vi "Scripting_ConnecorPaneCreateConstant.vi"(0 "ViRef":refnum<vi>, 1 "SubViThatHasChangedConnectorPane":path, 2 "ConnectorPaneIndexToCReateConstantsOn":u32[](array[numeric]), 5 "error in (no error)":errorcluster) -> (19 "error out":errorcluster)   [LabVIEW 2014]
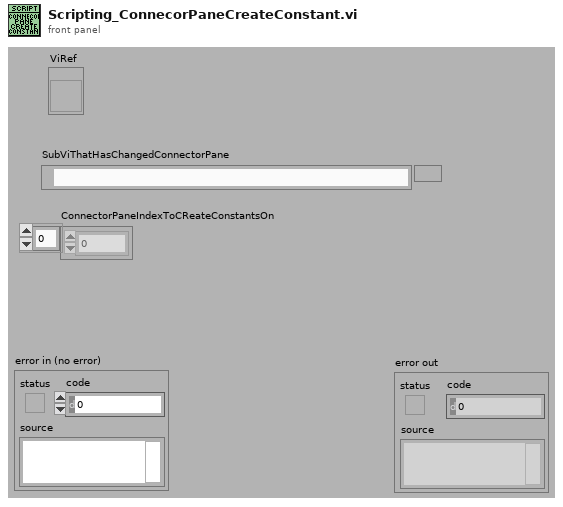
[diagram p1: front panel]
types:
  T1 = cluster{"New":refnum<vi>, "Terminals[]":refnum<vi>[]}
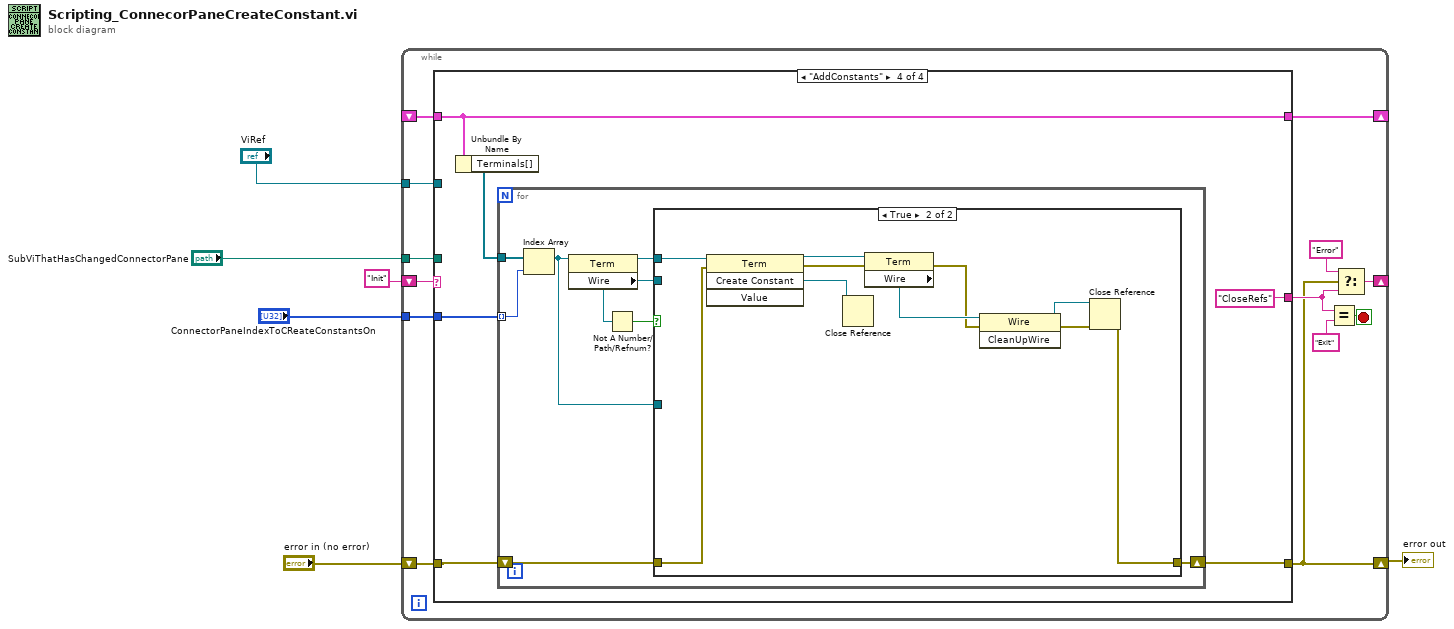
[diagram p0: block diagram]
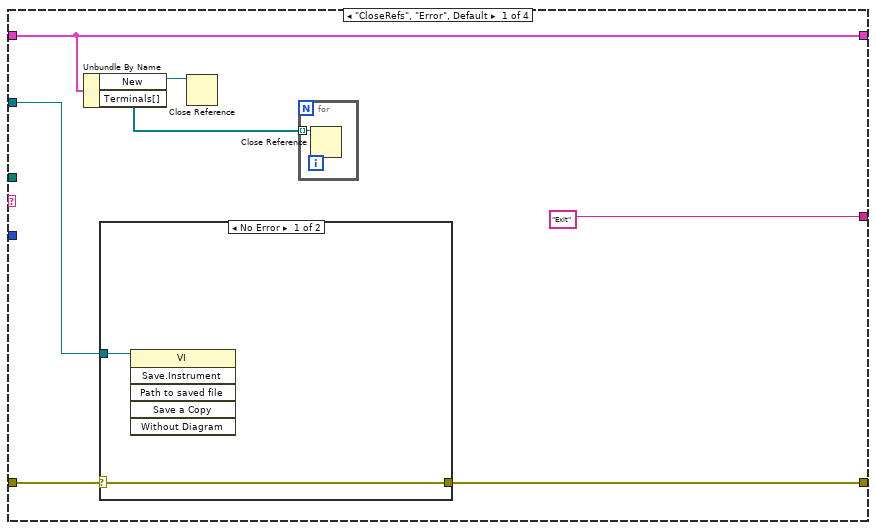
[diagram p2: hidden frame]
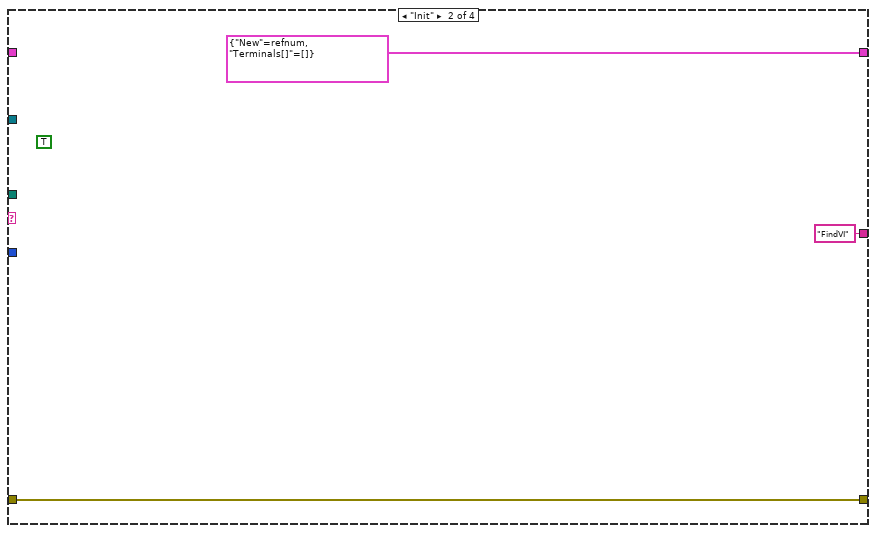
[diagram p4: hidden frame]
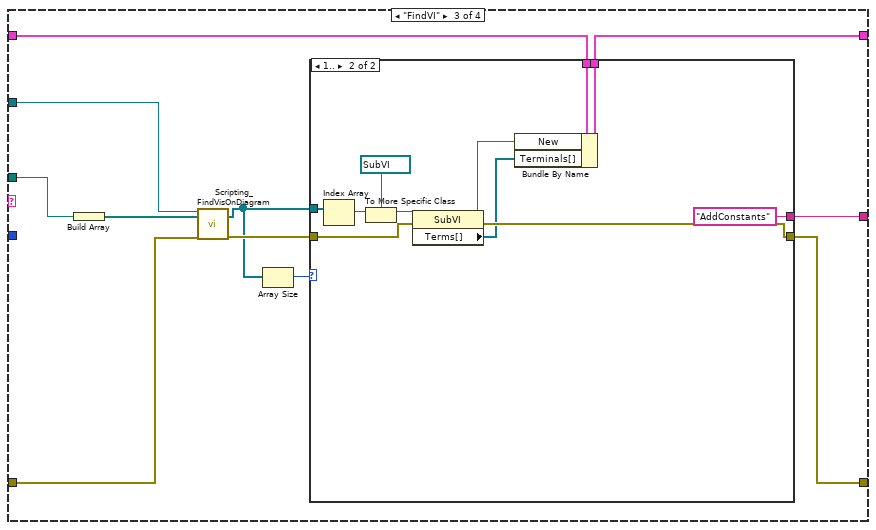
[diagram p5: hidden frame]
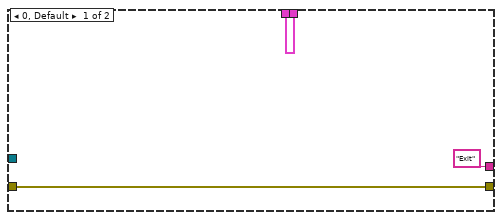
[diagram p6: hidden frame]
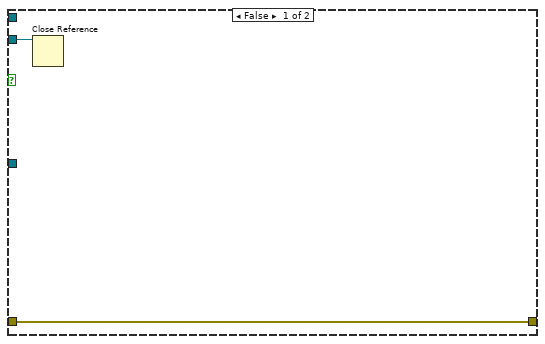
[diagram p7: hidden frame]
diagram:
  n1 = while {
    shift-right: [w12] -> w4
    shift-left: "error in (no error)" -> [w19]
    shift-right: [w17] -> _
    shift-left: "Init" -> [w18]
    shift-right: [w11] -> _
    shift-left: _ -> [w10]
    tunnel: "ViRef" -> [w9]
    tunnel: "SubViThatHasChangedConnectorPane" -> [w8]
    tunnel: "ConnectorPaneIndexToCReateConstantsOn" -> [w7]
    stop <- w16 stop-if-true
    n2 = case shown="\"AddConstants\"" w18 {
      tunnel: w19 -> [w24 w32 w43 w60]
      tunnel: [w23 w32 w35 w59] -> w12
      tunnel: ["Exit" "FindVI" w34 "CloseRefs"] -> w13
      tunnel: [w25 T1 {"New"=refnum, "Terminals[]"=[]} w38 w64] -> w11
      tunnel: w10 -> [w25 _ w39 w64]
      tunnel: w9 -> [w22 _ w42 _]
      tunnel: w8 -> [_ _ w41 _]
      tunnel: w7 -> [_ _ _ w61]
      frame "CloseRefs", "Error", Default {
        n3 = Unbundle By Name(w25) -> ("New"=w20:refnum<vi>, "Terminals[]"=w21:refnum<vi>[])
        n4 = case shown="No Error" w24 {
          selector: w24 -> [w28 w30]
          tunnel: [w28 w30] -> w23
          tunnel: w22 -> [w29 _]
          frame No Error {
            n5 = invoke class="VI" method="Save.Instrument"(reference=w29) -> ()  [unwired: 5 in, 6 out]
          }
          frame Error {
          }
        }
        n6 = Close Reference(reference=w20) -> ()  [unwired: 1 in, 1 out]
        n7 = for {
          tunnel: w21 -> [w27] mode=indexing
          n8 = Close Reference(reference=w27) -> ()  [unwired: 1 in, 1 out]
        }
      }
      frame "Init" {
        (unwired) TRUE ("Execution:Is Reentrant")
      }
      frame "FindVI" {
        n9 = Build Array(w41) -> (w40:path[])
        n10 = call <resource>:"Scripting_FindVisOnDiagram.vi"("ViRef"=w42, "VIsToSerachFor/ViName"=w40, "error in (no error)"=w43) -> ("VisFound"=w37:refnum<vi>[], "error out"=w44:errorcluster)  [unwired: 15 in]
        n11 = Array Size(array=w37) -> (size(s)=w36:i32)
        n12 = case shown="1.." w36 {
          tunnel: w44 -> [w46 w56]
          tunnel: w39 -> [w47 w54]
          tunnel: [w47 w53] -> w38
          tunnel: w37 -> [_ w52]
          tunnel: [w46 w51] -> w35
          tunnel: ["Exit" "AddConstants"] -> w34
          frame 0, Default {
          }
          frame 1.. {
            n13 = Index Array(array=w52) -> (element=w58:refnum<vi>)  [unwired: 1 in]
            n14 = To More Specific Class(target class=refnum<vi> refnum ("WhileLoop"), reference=w58) -> (specific class reference=w57:refnum<vi>)  [unwired: 1 in, 1 out]
            n15 = property class="SubVI"(reference=w57, error in=w56) -> (reference out=w50:refnum<vi>, error out=w51:errorcluster, "Terms[]"=w49:refnum<vi>[])
            n16 = Bundle By Name(cluster=w54, "New"=w50, "Terminals[]"=w49) -> (w53:T1)
          }
        }
      }
      frame "AddConstants" {
        n17 = Unbundle By Name(w64) -> ("Terminals[]"=w62:refnum<vi>[])
        n18 = for {
          tunnel: w62 -> [w68]
          tunnel: w61 -> [w72] mode=indexing
          shift-right: [w70] -> w59
          shift-left: w60 -> [w71]
          n19 = Index Array(array=w68, index=w72) -> (element=w69:refnum<vi>)
          n20 = property class="Term"(reference=w69) -> (reference out=w66:refnum<vi>, "Wire"=w65:refnum<vi>)  [unwired: 1 in, 1 out]
          n21 = Not A Number/Path/Refnum?(number/path/refnum=w65) -> (NaN/Path/Refnum?=w67:bool)
          n22 = case shown="True" w67 {
            tunnel: w71 -> [w74 w76]
            tunnel: [w74 w81] -> w70
            tunnel: w69 -> [_ _]
            tunnel: w66 -> [_ w80]
            tunnel: w65 -> [w73 _]
            frame False {
              n23 = Close Reference(reference=w73) -> ()  [unwired: 1 in, 1 out]
            }
            frame True {
              n24 = invoke class="Term" method="Create Constant"(reference=w80, error in=w76) -> (reference out=w79:refnum<vi>, error out=w78:errorcluster, "Create Constant"=w75:refnum<vi>)  [unwired: 2 in, 1 out]
              n25 = Close Reference(reference=w75) -> ()  [unwired: 1 in, 1 out]
              n26 = property class="Term"(reference=w79, error in=w78) -> (error out=w77:errorcluster, "Wire"=w84:refnum<vi>)  [unwired: 1 out]
              n27 = invoke class="Wire" method="CleanUpWire"(reference=w84, error in=w77) -> (reference out=w82:refnum<vi>, error out=w83:errorcluster)  [unwired: 1 in, 1 out]
              n28 = Close Reference(reference=w82, error in (no error)=w83) -> (error out=w81:errorcluster)
            }
          }
        }
      }
    }
    n29 = Equal?(x=w13, y="Exit") -> (x = y?=w16:bool)
    n30 = Select(t="Error", s=w12, f=w13) -> (s? t:f=w17:string)
  }
  "error out" <- w4
